vi "Error Handler.vi"(8 "error in (no error)":errorcluster, 11 "other error":errorcluster) -> (0 "error out":errorcluster, 3 "stop program?":bool)   [LabVIEW 2020]
uses:
  <vilib>/Utility/error.llb/DialogType.ctl
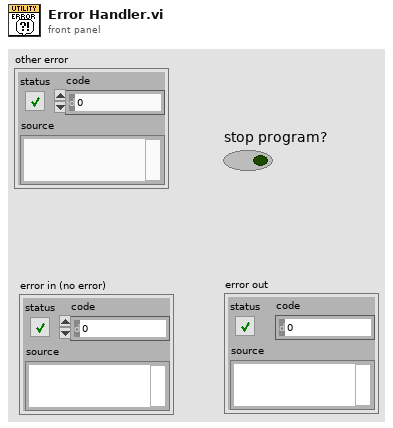
[diagram p1: front panel]
types:
  T1 = typedef "DialogType.ctl" = u16
  T2 = enum16{"Left Button", "Center Button", "Right Button", "Window Close"}
  T3 = enum32{"invalid app kind", "Development System", "Run Time System", "Student Edition", "Embedded LabVIEW", "Evaluation", "Custom"}
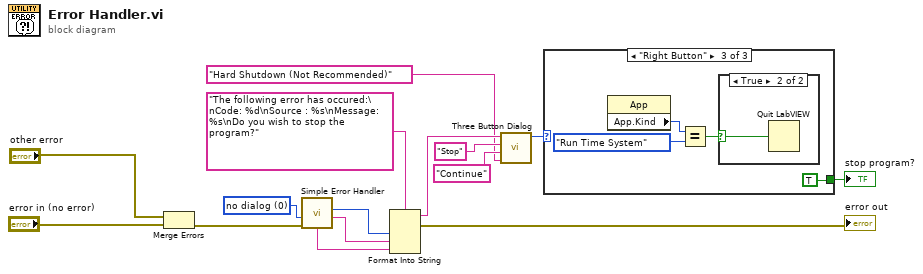
[diagram p0: block diagram]
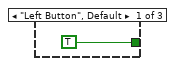
[diagram p2: hidden frame]
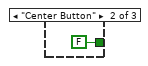
[diagram p3: hidden frame]
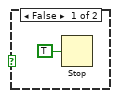
[diagram p4: hidden frame]
diagram:
  w11 = T1 0 items=["no dialog", "OK message", "continue or stop message", "OK message + warnings", "continue/stop + warnings"] ("type of dialog (OK msg:1)")
  n1 = Merge Errors("other error", "error in (no error)") -> (w8:errorcluster)
  n2 = call <vilib>:"Simple Error Handler.vi"("type of dialog (OK msg:1)"=w11, "error in (no error)"=w8) -> ("code out"=w12:i32, "source out"=w13:string, "message"=w15:string)  [unwired: 3 in, 2 out]
  n3 = Format Into String(format string="The following error has occured:\nCode: %d\nSource : %s\nMessage: %s\nDo you wish to stop the program?", w12, w13, w15) -> (resulting string=w4:string, error out=→"error out":errorcluster)  [unwired: 2 in]
  n4 = call <vilib>:"Three Button Dialog.vi"("Right Button Text (\"Cancel\")"="Hard Shutdown (Not Recommended)" ("Right Button Text (\"Cancel\")"), "Center Button Text (\"No\")"="Continue" ("F button name (\"Cancel\")"), "Left Button Text (\"Yes\")"="Stop" ("T button name (\"OK\")"), "message"=w4) -> ("Which Button?"=w3:T2)  [unwired: 7 in]
  n5 = case shown="\"Right Button\"" w3 {
    tunnel: [TRUE ("stop program?") FALSE ("stop program?") TRUE ("stop program?")] -> w1
    frame "Left Button", Default {
    }
    frame "Center Button" {
    }
    frame "Right Button" {
      n6 = property class="App"() -> ("App.Kind"=w19:T3)  [unwired: 2 in, 2 out]
      n7 = Equal?(x=w19, y=T3."Run Time System" ("Application:Kind")) -> (x = y?=w20:bool)
      n8 = case shown="True" w20 {
        selector: w20 -> [_ w23]
        frame False {
          n9 = Stop(stop? (T)=TRUE) -> ()
        }
        frame True {
          n10 = Quit LabVIEW(quit? (T)=w23) -> ()
        }
      }
    }
  }
  "stop program?" <- w1
